vi "LoggingLoop.vi"(8 "Error In":errorcluster, 11 "Communication References":T1) -> (0 "Error Out":errorcluster)   [LabVIEW 2017, in "Client.lvlib" / "ClientLogger.lvlib"]
doc: "This Loop accepts \"Log\"-Messages with LogData.ctl as Datatype. It then logs the Type of Message, the Message Data and the Timestamp of the message to a tdms-file."
uses:
  ClientLogger.lvlib
  Error Cluster From Error Code.vi
  Error Ring.xnode
  Message Queue.lvlib
  ClientErrorHandler.lvlib
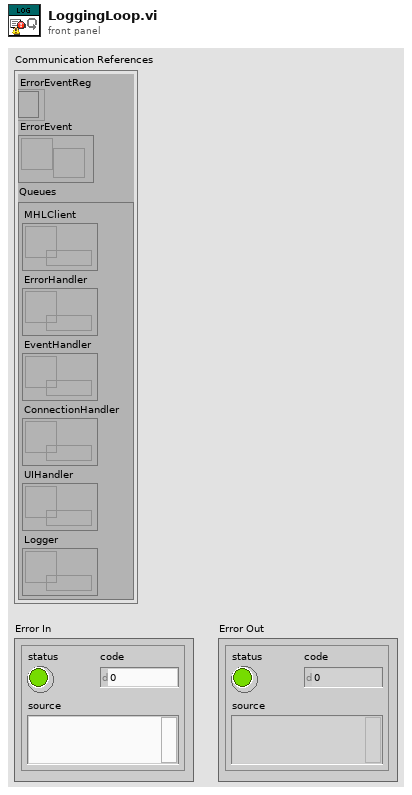
[diagram p1: front panel]
types:
  T1 = cluster{"ErrorEventReg":refnum<event-registration>, "ErrorEvent":refnum<user-event>, "Queues":cluster{"MHLClient":refnum<queue>, "ErrorHandler":refnum<queue>, "EventHandler":refnum<queue>, "ConnectionHandler":refnum<queue>, "UIHandler":refnum<queue>, "Logger":refnum<queue>}}
  T2 = enum16{"open", "open or create", "create or replace", "create", "open (read-only)"}
  T3 = cluster{"ClientTimeout (s)":u32, "LogPath":path, "ErrorsToIgnore":i32[], "OracleData":cluster{"DBname":string, "User":string, "Password":string}}
  T4 = cluster{"Time":timestamp, "Type":string, "LogText":string}
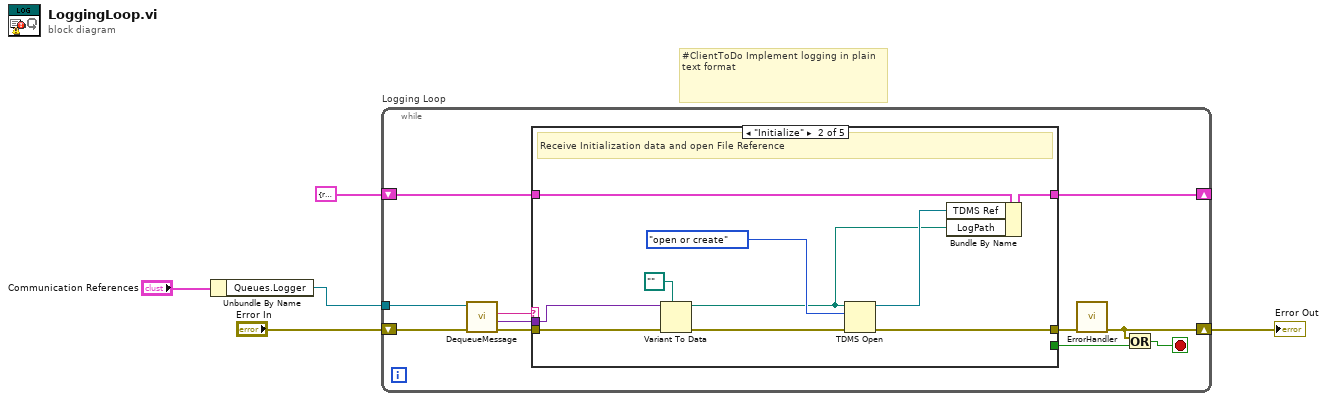
[diagram p0: block diagram]
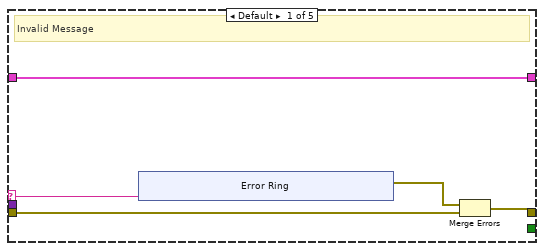
[diagram p2: hidden frame]
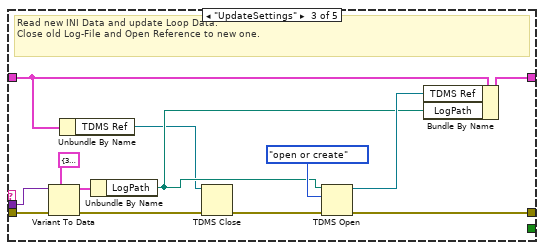
[diagram p3: hidden frame]
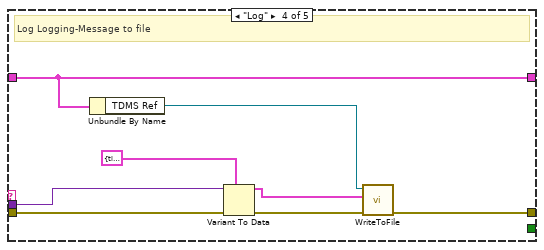
[diagram p4: hidden frame]
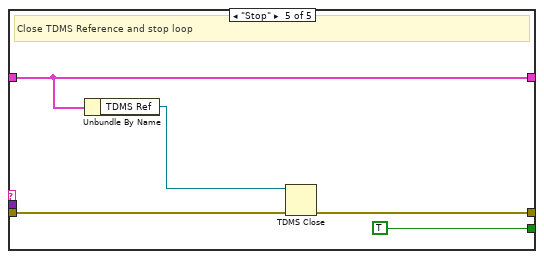
[diagram p5: hidden frame]
diagram:
  # "#ClientToDo Implement logging in plain text format"
  n1 = Unbundle By Name("Communication References") -> ("Queues.Logger"=w3:refnum<queue>)
  n2 = while "Logging Loop" {
    shift-right: [w7] -> w4
    shift-left: "Error In" -> [w16]
    tunnel: w3 -> [w6]
    shift-right: [w10] -> _
    shift-left: cluster{"TDMS Ref":refnum<k34>, "LogPath":path} {"TDMS Ref"=refnum, "LogPath"=path ""} ("LoggingLoopData") -> [w11]
    stop <- w9 stop-if-true
    n3 = call "DequeueMessage.vi"("error in (no error)"=w16, "Message Queue"=w6) -> ("error out"=w15:errorcluster, "Message Data"=w13:variant, "Message"=w14:string)  [unwired: 5 in, 2 out]
    n4 = case shown="\"Initialize\"" w14 {
      selector: w14 -> [w20 _ _ _ _]
      tunnel: [w19 w37 w50 w55 w62] -> w8
      tunnel: w15 -> [w21 w38 w51 w59 w64]
      tunnel: w13 -> [_ w33 w47 w57 _]
      tunnel: [_ _ _ _ TRUE] -> w12
      tunnel: [w17 w32 w45 w53 w61] -> w10
      tunnel: w11 -> [w17 w35 w41 w53 w61]
      frame Default {
        # "Invalid Message"
        n5 = xnode "Error Ring"("parameter 0"=w20) -> ("error out"=w18:errorcluster)
        n6 = Merge Errors(w18, w21) -> (w19:errorcluster)
      }
      frame "Initialize" {
        # "Receive Initialization data and open File Reference"
        n7 = Variant To Data(error in=w38, type=path "", Variant=w33) -> (data=w29:path, error out=w34:errorcluster)
        n8 = TDMS Open(8:w34, 10:T2."open or create" ("operation (0:open)"), 11:w29) -> (0:w37:errorcluster, 3:w31:refnum<k34>)  [unwired: 4 in]
        n9 = Bundle By Name(cluster=w35, "TDMS Ref"=w31, "LogPath"=w29) -> (w32:cluster{"TDMS Ref":refnum<k34>, "LogPath":path})
      }
      frame "UpdateSettings" {
        # "Read new INI Data and update Loop Data.\nClose old Log-File and Open Reference to new one."
        n10 = Variant To Data(error in=w51, type=T3 {"ClientTimeout (s)"=30, "LogPath"=path "C:/Users/jgoebel/Documents/GitHub/AEDashboard/ServerLib/Data/ServerLog.tdms", "ErrorsToIgnore"=[], "OracleData"={"DBname"="", "User"="", "Password"=""}} ("ServerINI"), Variant=w47) -> (data=w43:T3, error out=w48:errorcluster)
        n11 = Unbundle By Name(w41) -> ("TDMS Ref"=w39:refnum<k34>)
        n12 = Unbundle By Name(w43) -> ("LogPath"=w42:path)
        n13 = TDMS Close(8:w48, 11:w39) -> (0:w40:errorcluster)  [unwired: 1 out]
        n14 = TDMS Open(8:w40, 10:T2."open or create" ("operation (0:open)"), 11:w42) -> (0:w50:errorcluster, 3:w44:refnum<k34>)  [unwired: 4 in]
        n15 = Bundle By Name(cluster=w41, "TDMS Ref"=w44, "LogPath"=w42) -> (w45:cluster{"TDMS Ref":refnum<k34>, "LogPath":path})
      }
      frame "Log" {
        # "Log Logging-Message to file"
        n16 = Unbundle By Name(w53) -> ("TDMS Ref"=w52:refnum<k34>)
        n17 = Variant To Data(error in=w59, type=T4 {"Time"=timestamp(0 s since 1904-01-01), "Type"="", "LogText"=""} ("LogData"), Variant=w57) -> (data=w54:T4, error out=w58:errorcluster)
        n18 = call "WriteToFile.vi"("error in (no error)"=w58, "LogData"=w54, "Refnum in"=w52) -> ("error out"=w55:errorcluster)  [unwired: 7 in, 1 out]
      }
      frame "Stop" {
        # "Close TDMS Reference and stop loop"
        n19 = Unbundle By Name(w61) -> ("TDMS Ref"=w60:refnum<k34>)
        n20 = TDMS Close(8:w64, 11:w60) -> (0:w62:errorcluster)  [unwired: 1 out]
      }
    }
    n21 = call "ErrorHandler.vi"("error in (no error)"=w8) -> ("error out"=w7:errorcluster)  [unwired: 10 in]
    n22 = Or(x=w7, y=w12) -> (x .or. y?=w9:bool)
  }
  "Error Out" <- w4
